vi "IMAQ-GetContrast.vi"(5 "Image Device IN":cluster{"Image":T1, "errorImage":errorcluster}) -> (1 "RMS Contraste":dbl format="%.2f", 2 "Image Device OUT":cluster{"Image":T1, "errorImage":errorcluster})   [LabVIEW 2010]
uses:
  <vilib>/vision/Image Controls.llb/IMAQ Image.ctl
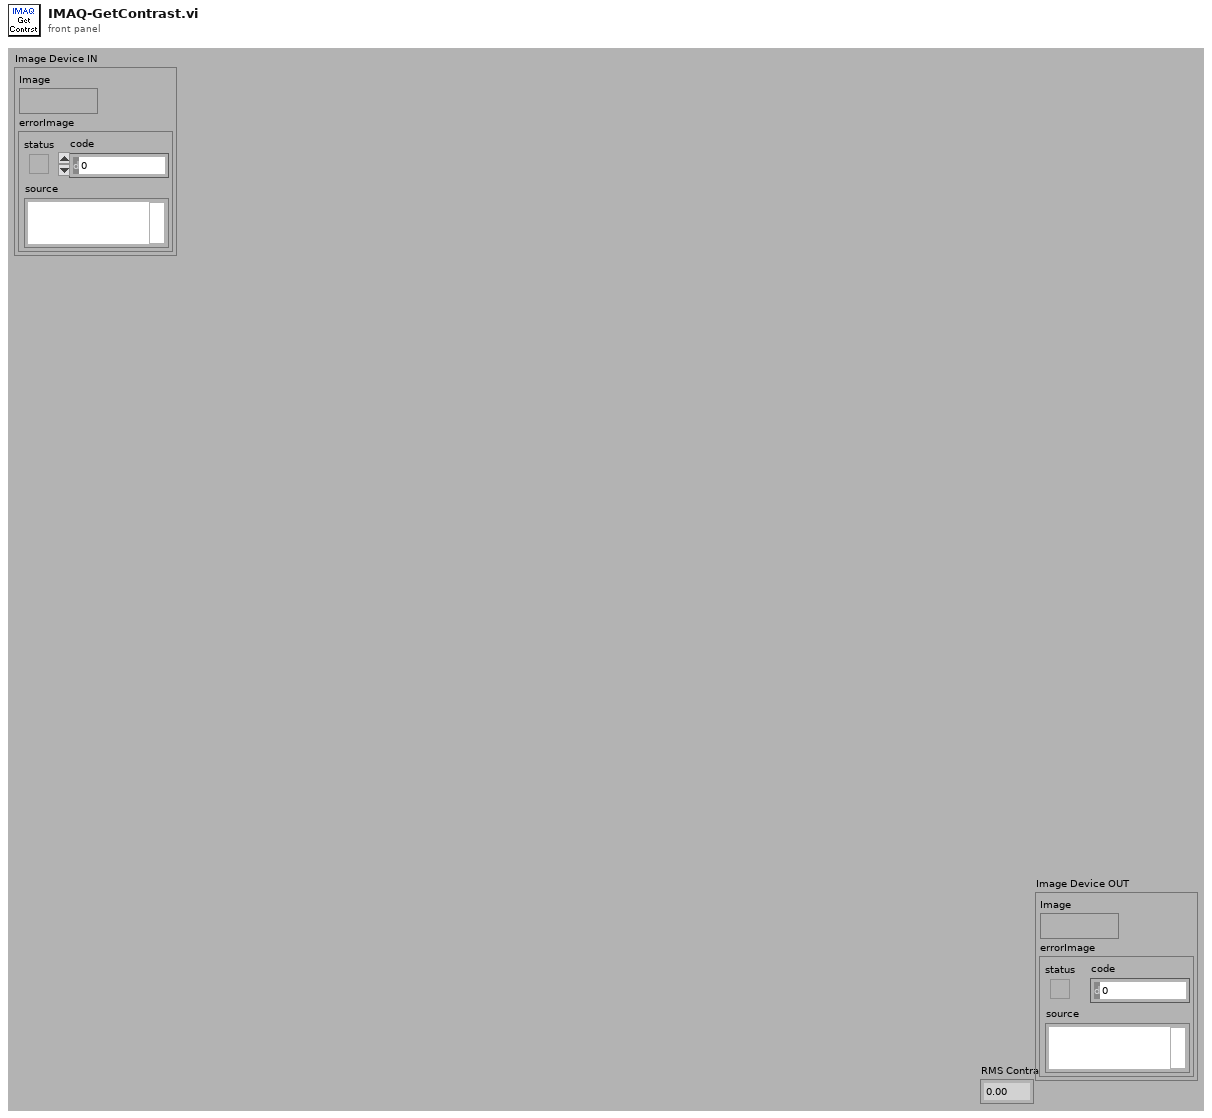
[diagram p1: front panel]
types:
  T1 = typedef "IMAQ Image.ctl" = refnum<image>
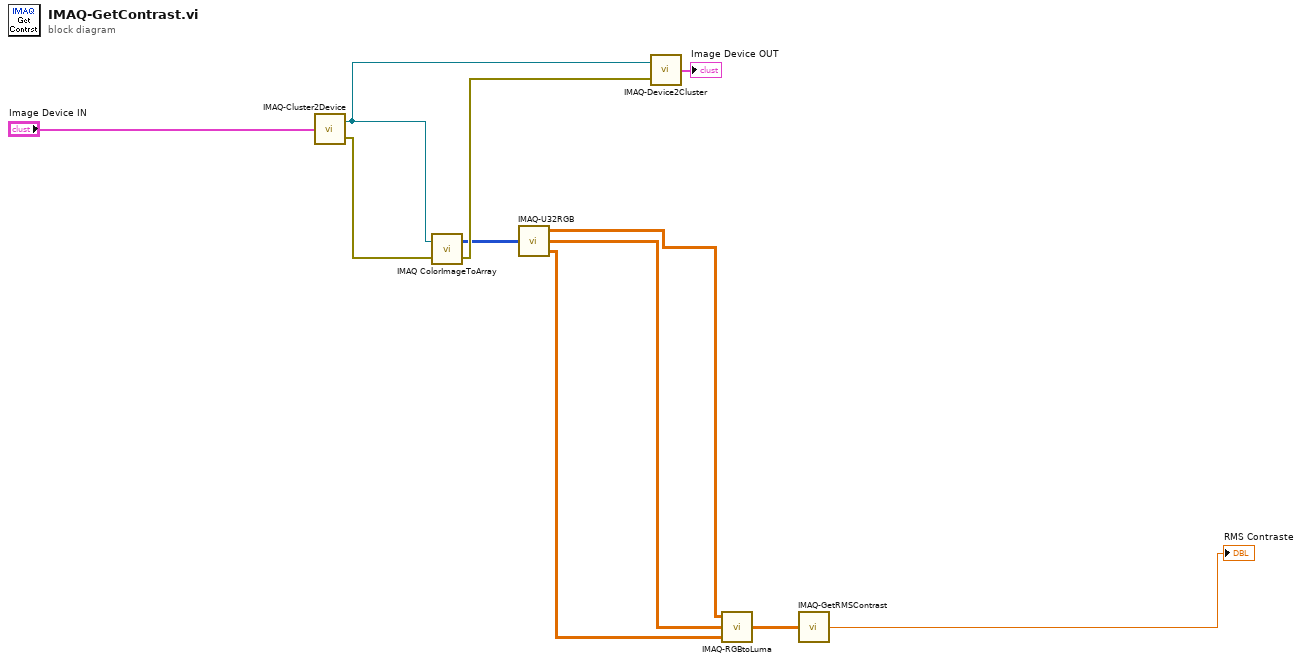
[diagram p0: block diagram]
diagram:
  n1 = call "IMAQ-Cluster2Device.vi"("Image Device IN"="Image Device IN") -> ("errorImage OUT"=w8:errorcluster, "Image OUT"=w9:T1)
  n2 = call "IMAQ ColorImageToArray"("Image"=w9, "error in (no error)"=w8) -> ("Image Pixels (U32)"=w6:u32[][], "error out"=w7:errorcluster)  [unwired: 2 in, 1 out]
  n3 = call "IMAQ-U32RGB.vi"("Image Pixels (RGB32) 2D Array"=w6) -> ("Blue 2D Array"=w3:dbl[][], "Green 2D Array"=w4:dbl[][], "Red 2D Array"=w5:dbl[][])
  n4 = call "IMAQ-Device2Cluster.vi"("errorImage IN"=w7, "Image IN"=w9) -> ("Image Device OUT"=→"Image Device OUT":cluster{"Image":T1, "errorImage":errorcluster})
  n5 = call "IMAQ-RGBtoLuma.vi"("Blue 2D Array"=w3, "Green 2D Array"=w4, "Red 2D Array"=w5) -> ("Luma 2D Array"=w2:dbl[][])
  n6 = call "IMAQ-GetRMSContrast.vi"("Intensity 2D Array"=w2) -> ("RMS Contrast"=→"RMS Contraste":dbl)
